vi "svx_Timebase Manage Grid.vi"(4 "Minor Color":u32, 6 "Major Color":u32, 7 "Axis":enum16{"X-Scale", "Y-Scale", "Z-Scale"}(ring), 9 "Grid Style":u16, 10 "Probe Y in":refnum<vi>, 11 "Probe X in":refnum<vi>) -> (0 "Minor Disabled":u8, 1 "Major Disabled":u8, 2 "Probe Y out":refnum<vi>, 3 "Probe X out":refnum<vi>)   [LabVIEW 2017, in "SVX Timebase.xctl"]
uses:
  <vilib>/addons/_XControls/Timebase Plot/SVX Timebase.xctl
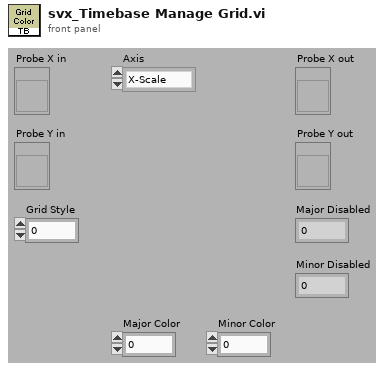
[diagram p1: front panel]
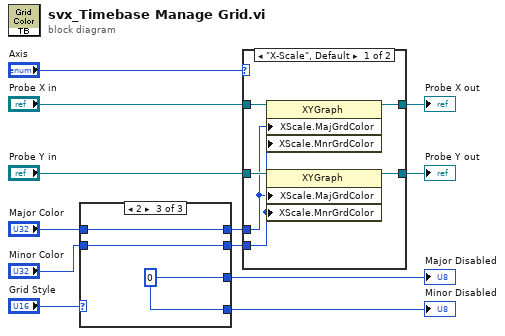
[diagram p0: block diagram]
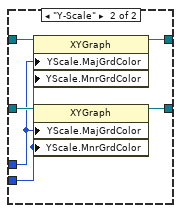
[diagram p2: hidden frame]
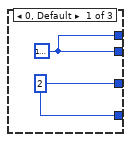
[diagram p3: hidden frame]
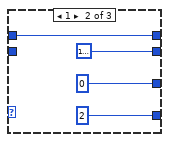
[diagram p4: hidden frame]
diagram:
  n1 = case shown="2" "Grid Style" {
    tunnel: [w14 u8 0 ("Disabled") w21] -> w10
    tunnel: [w14 u8 2 ("Disabled") w21] -> w9
    tunnel: [w13 w15 w20] -> w2
    tunnel: [w13 u32 16777216 w19] -> w8
    tunnel: "Major Color" -> [_ w15 w20]
    tunnel: "Minor Color" -> [_ _ w19]
    frame 0, Default {
      w13 = u32 16777216
      w14 = u8 2 ("Disabled")
    }
    frame 1 {
    }
    frame 2 {
      w21 = u8 0 ("Disabled")
    }
  }
  "Major Disabled" <- w10
  "Minor Disabled" <- w9
  n2 = case shown="\"X-Scale\", Default" "Axis" {
    tunnel: "Probe X in" -> [w27 w33]
    tunnel: w8 -> [w24 w29]
    tunnel: [w26 w32] -> w4
    tunnel: "Probe Y in" -> [w25 w31]
    tunnel: w2 -> [w23 w30]
    tunnel: [w22 w28] -> w1
    frame "X-Scale", Default {
      n3 = property class="XYGraph"(reference=w27, "XScale.MajGrdColor"=w23, "XScale.MnrGrdColor"=w24) -> (reference out=w26:refnum<vi>)  [unwired: 1 in, 1 out]
      n4 = property class="XYGraph"(reference=w25, "XScale.MajGrdColor"=w23, "XScale.MnrGrdColor"=w24) -> (reference out=w22:refnum<vi>)  [unwired: 1 in, 1 out]
    }
    frame "Y-Scale" {
      n5 = property class="XYGraph"(reference=w33, "YScale.MajGrdColor"=w30, "YScale.MnrGrdColor"=w29) -> (reference out=w32:refnum<vi>)  [unwired: 1 in, 1 out]
      n6 = property class="XYGraph"(reference=w31, "YScale.MajGrdColor"=w30, "YScale.MnrGrdColor"=w29) -> (reference out=w28:refnum<vi>)  [unwired: 1 in, 1 out]
    }
  }
  "Probe X out" <- w4
  "Probe Y out" <- w1
